vi "Read Type.vi"(8 "error in (no error)":errorcluster, 11 "Instruction in":refnum<class "Instruction.lvclass">) -> (0 "error out":errorcluster, 2 "Type":string, 3 "Instruction out":refnum<class "Instruction.lvclass">)   [LabVIEW 2015, in "Instruction.lvclass"]
uses:
  Instruction.lvclass
  Instruction.lvclass/Instruction.ctl
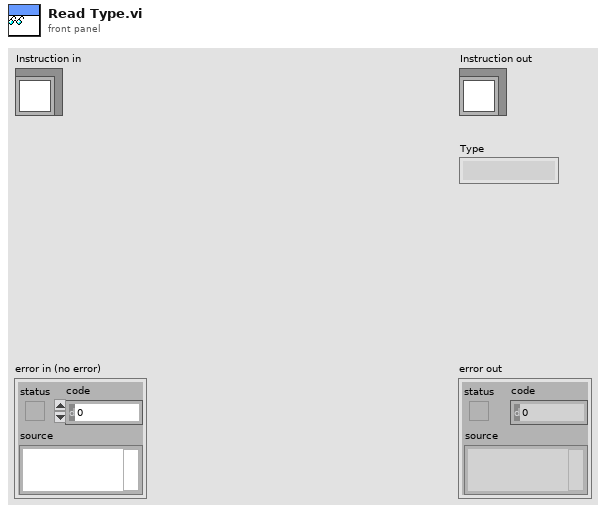
[diagram p1: front panel]
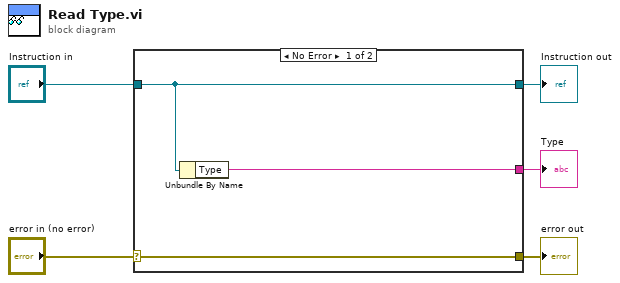
[diagram p0: block diagram]
diagram:
  n1 = case shown="No Error" "error in (no error)" {
    selector: "error in (no error)" -> [w8 w9]
    tunnel: [w8 w9] -> w4
    tunnel: [w7 w10] -> w2
    tunnel: "Instruction in" -> [w7 w10]
    tunnel: [w6 _] -> w1
    frame No Error {
      n2 = Unbundle By Name(w7) -> ("Type"=w6:string)
    }
    frame Error {
    }
  }
  "error out" <- w4
  "Instruction out" <- w2
  "Type" <- w1
